vi "4_2.vi"() -> ()   [LabVIEW 2012]
panel:
  in  "stop":bool
  in  "OK Button":bool
  in  "String":string
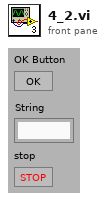
[diagram p1: front panel]
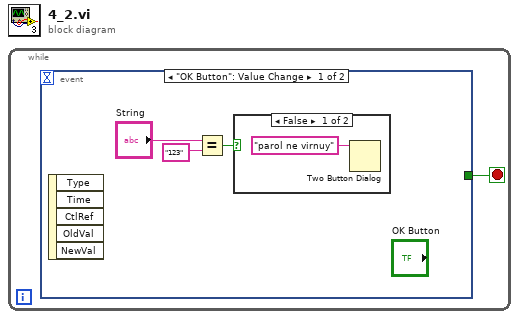
[diagram p0: block diagram]
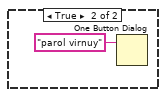
[diagram p2: hidden frame]
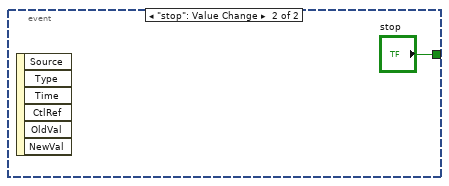
[diagram p3: hidden frame]
diagram:
  n1 = while {
    stop <- w1 stop-if-true
    n2 = event shown="[0] \"OK Button\": Value Change" {
      selector: _ -> [_ _]
      dyn-events: _ -> [_ _]
      timeout: _ -> [_ _]
      tunnel: [_ "stop"] -> w1
      event "OK Button": Value Change {
        n3 = event-data() -> ()  [unwired: 1 in, 5 out]
        n4 = Equal?(x="String", y="123") -> (x = y?=w2:bool)
        n5 = case shown="False" w2 {
          frame False {
            n6 = Two Button Dialog(message="parol ne virnuy") -> ()  [unwired: 2 in, 1 out]
          }
          frame True {
            n7 = One Button Dialog(message="parol virnuy") -> ()  [unwired: 2 out]
          }
        }
      }
      event "stop": Value Change {
        n8 = event-data() -> ()  [unwired: 1 in, 6 out]
      }
    }
  }
